vi "prot version global.vi"() -> ()   [LabVIEW 2018, in "LV2Julia_core.lvlib"]
uses:
  LV2Julia_core.lvlib
panel:
  out "PROTOC_V":u8=1
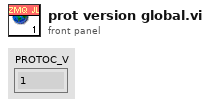
[diagram p1: front panel]
diagram:
